vi "Get Collection Subtype__ogtk.vi"(7 "Type Descriptor":T1, 10 "Offset In":i16) -> (0 "Size":i16, 1 "subtype":T1, 2 "Offset out":i16)   [LabVIEW 2023, in "openg_variant.lvlib"]
uses:
  openg_variant.lvlib
  Type Descriptor__ogtk.ctl
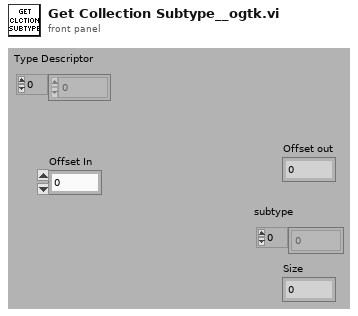
[diagram p1: front panel]
types:
  T1 = typedef "openg_variant.lvlib/Type Descriptor__ogtk.ctl" = i16[]
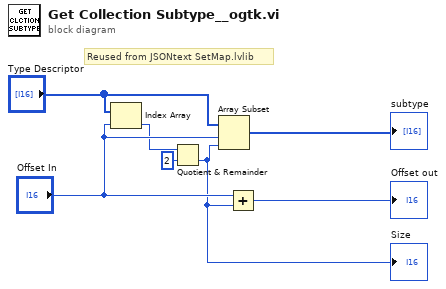
[diagram p0: block diagram]
diagram:
  # "Reused from JSONtext SetMap.lvlib"
  n1 = Index Array(array="Type Descriptor", index="Offset In") -> (element=w3:i16)
  n2 = Quotient & Remainder(x=w3, y=i16 2) -> (floor(x/y)=w2:i16)  [unwired: 1 out]
  "Size" <- w2
  n3 = Array Subset(array="Type Descriptor", index="Offset In", length=w2) -> (→"subtype":T1)
  n4 = Add(x="Offset In", y=w2) -> (x+y=→"Offset out":i16)
